vi "请求注销.vi"(8 "error in (no error)":errorcluster caption="错误输入（无错误）", 10 "数据采集.lvclass":refnum<class "数据采集.lvclass">, 11 "数据显示 输入":refnum<class "数据显示.lvclass"> caption="DNL_LabVIEW Object in") -> (0 "error out":errorcluster caption="错误输出", 3 "数据显示 输出":refnum<class "数据显示.lvclass"> caption="DNL_LabVIEW Object out")   [LabVIEW 2011, in "数据显示.lvclass"]
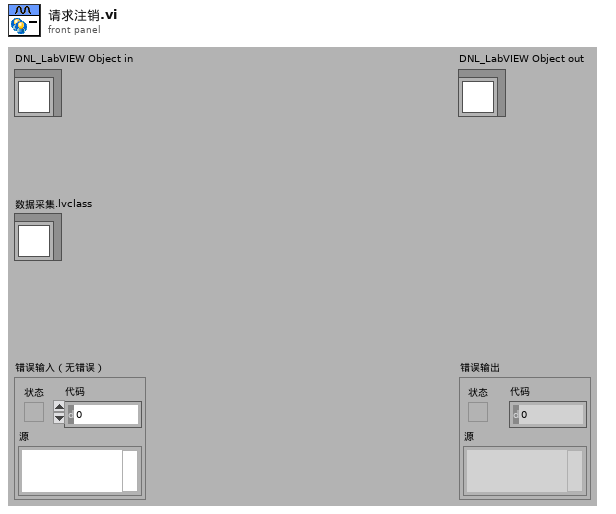
[diagram p1: front panel]
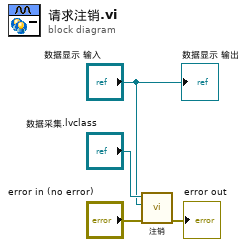
[diagram p0: block diagram]
diagram:
  n1 = call-dynamic "注销.vi"("error in (no error)"="error in (no error)", "数据值引用"="数据显示 输入", "数据采集 输入"="数据采集.lvclass") -> ("error out"=→"error out":errorcluster)  [unwired: 7 in, 1 out]
  "数据显示 输出" <- "数据显示 输入"
